vi "json_api.vi"() -> ()   [LabVIEW 2020]
uses:
  <vilib>/httpClient/LabVIEWHTTPClient.lvlib
panel:
  out "value":T1(array[cluster])
  in  "Array":T1(array[cluster])
  in  "stop":bool
  out "body":string
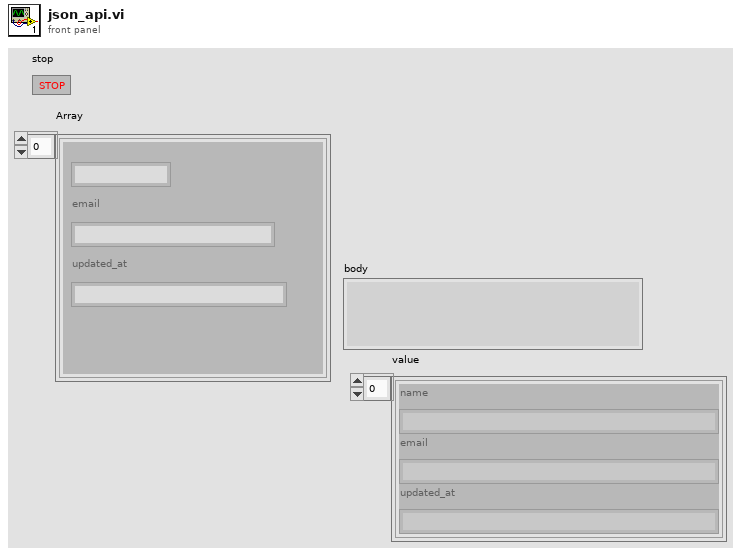
[diagram p1: front panel]
types:
  T1 = cluster{"name":string, "email":string, "updated_at":string}[]
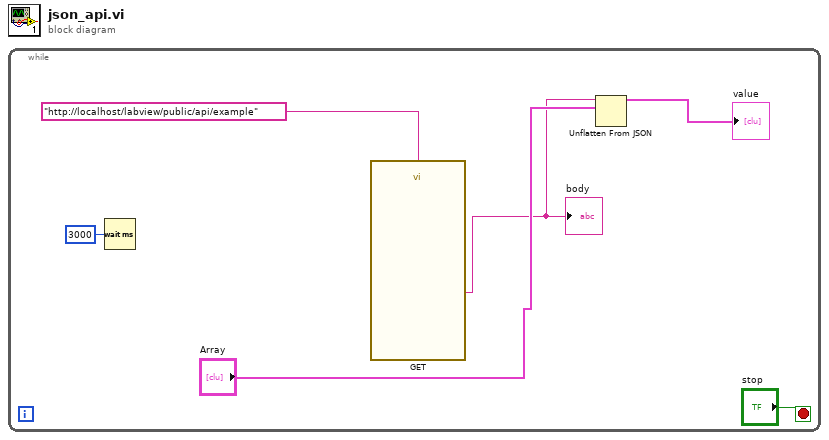
[diagram p0: block diagram]
diagram:
  n1 = while {
    stop <- "stop" stop-if-true
    n2 = Wait (ms)(milliseconds to wait=u32 3000) -> ()  [unwired: 1 out]
    n3 = call <vilib>:"GET.vi"("url"="http://localhost/labview/public/api/example") -> ("body"=w2:string)  [unwired: 11 in, 3 out]
    "body" <- w2
    n4 = Unflatten From JSON(JSON string=w2, type and defaults="Array") -> (value=→"value":T1)  [unwired: 5 in, 1 out]
  }
